vi "test_0.1.0a1.vi"() -> ()   [LabVIEW 2011]
uses:
  bin/libctiff.dll
panel:
  in  "path in":path=path "\\\\vmware-host\\Shared Folders/shared/camtiff/bin/libctiff.dll"
  out "error out":errorcluster
  in  "meta":string="{\"data to add\" : 1}"
  in  "name":string="LabVIEW"
  in  "image_desc":string="LabVIEW Testing"
  in  "software":string="Make"
  in  "model":string="Model"
  in  "make":string="Make"
  in  "copyright":string="Copyright"
  in  "artist":string="Artist"
  in  "output_file":string="labview_test.tiff"
  in  "Array":u16[][](array[numeric])=[[0, 0, 0, 0], [0, 24000, 0, 0], [0, 0, 37000, 0], [0, 0, 0, 65535]]
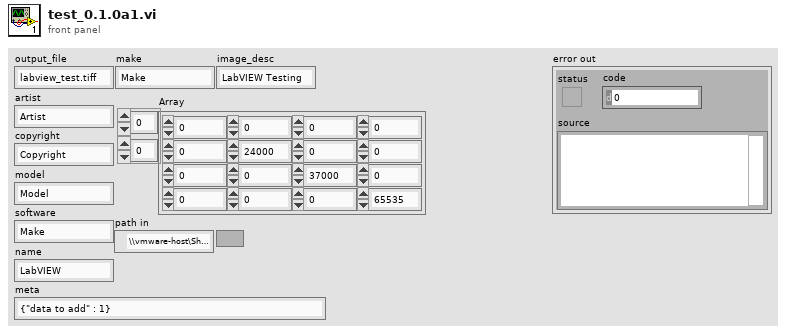
[diagram p1: front panel]
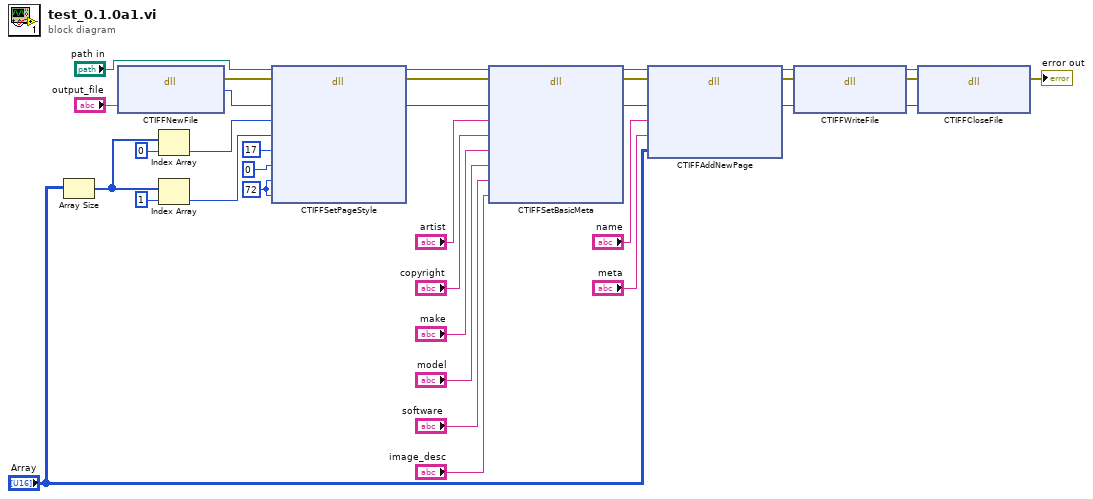
[diagram p0: block diagram]
diagram:
  w17 = u32 72 ("x_resolution")
  n1 = Array Size(array="Array") -> (size(s)=w23:i32[])
  n2 = dll-call lib="\\\\vmware-host\\Shared Folders/shared/camtiff/bin/libctiff.dll" fn="CTIFFNewFile"("output_file"="output_file") -> (error out=w9:errorcluster, "return type"=w25:i64)  [unwired: 4 in, 1 out]
  n3 = Index Array(array=w23, index=0) -> (element=w21:i32)
  n4 = Index Array(array=w23, index=1) -> (element=w20:i32)
  n5 = dll-call lib="?" fn="CTIFFSetPageStyle"(path in="path in", error in=w9, "ctiff"=w25, "width"=w21, "height"=w20, "pixel_type"=u32 17, "in_color"=u8 0, "x_resolution"=w17, "y_resolution"=w17) -> (path out=w27:path, error out=w10:errorcluster, "ctiff"=w26:i64)  [unwired: 8 in]
  n6 = dll-call lib="?" fn="CTIFFSetBasicMeta"(path in=w27, error in=w10, "ctiff"=w26, "artist"="artist", "copyright"="copyright", "make"="make", "model"="model", "software"="software", "image_desc"="image_desc") -> (path out=w12:path, error out=w11:errorcluster, "ctiff"=w16:i64)  [unwired: 8 in]
  n7 = dll-call lib="?" fn="CTIFFAddNewPage"(path in=w12, error in=w11, "ctiff"=w16, "name"="name", "meta"="meta", "buffer"="Array") -> (path out=w8:path, error out=w7:errorcluster, "ctiff"=w6:i64)  [unwired: 5 in]
  n8 = dll-call lib="?" fn="CTIFFWriteFile"(path in=w8, error in=w7, "ctiff"=w6) -> (path out=w5:path, error out=w4:errorcluster, "ctiff"=w3:i64)  [unwired: 2 in]
  n9 = dll-call lib="?" fn="CTIFFCloseFile"(path in=w5, error in=w4, "ctiff"=w3) -> (error out=→"error out":errorcluster)  [unwired: 3 in, 1 out]
